vi "NI-XNET Frame&Log - CAN Frame to Table.vi"(1 "Hexadecimal?":bool, 5 "CAN Frames":T1[](array[typedef]) {"payload" format="%x"; "timestamp" format="%<%.7X\n%x>T"; "type" items=["CAN Data"=0, "CAN Remote"=1, "CAN Bus Error"=2, "Delay"=224, "Log Trigger"=225, "Start Trigger"=226]; "identifier" format="%x"}) -> (4 "Output Array":string[][](array[string]))   [LabVIEW 2014]
uses:
  <vilib>/xnet/xnet.llb/XNET Frame CAN.ctl
  <vilib>/xnet/xnet.llb/XNET Frame Type CAN.ctl
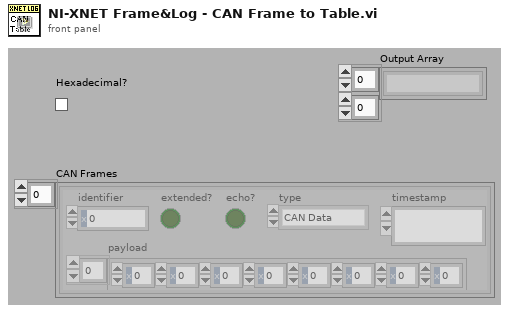
[diagram p1: front panel]
types:
  T1 = typedef "XNET Frame CAN.ctl" = cluster{"timestamp":timestamp, "payload":u8[], "identifier":u32, "type":T2, "extended?":bool, "echo?":bool}
  T2 = typedef "XNET Frame Type CAN.ctl" = u8
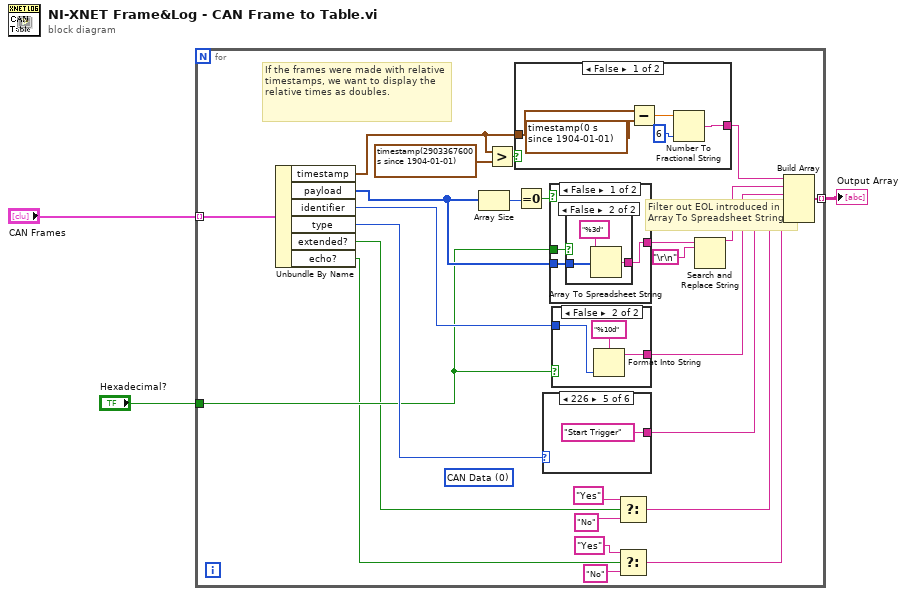
[diagram p0: block diagram]
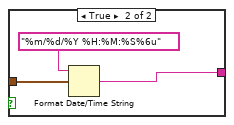
[diagram p2: hidden frame]
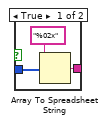
[diagram p3: hidden frame]
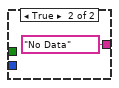
[diagram p4: hidden frame]
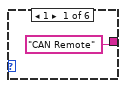
[diagram p5: hidden frame]
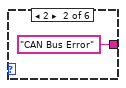
[diagram p6: hidden frame]
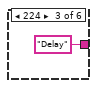
[diagram p7: hidden frame]
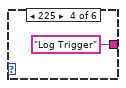
[diagram p8: hidden frame]
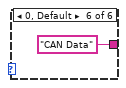
[diagram p9: hidden frame]
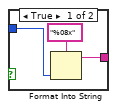
[diagram p10: hidden frame]
diagram:
  n1 = for {
    tunnel: "CAN Frames" -> [w28] mode=indexing
    tunnel: "Hexadecimal?" -> [w20]
    tunnel: [w19] -> w1 mode=indexing
    (unwired) T2 0 items=["CAN Data"=0, "CAN Remote"=1, "CAN Bus Error"=2, "Delay"=224, "Log Trigger"=225, "Start Trigger"=226] ("type")
    # "Filter out EOL introduced in \nArray To Spreadsheet String"
    # "If the frames were made with relative timestamps, we want to display the relative times as doubles."
    n2 = Unbundle By Name(w28) -> ("timestamp"=w10:timestamp, "payload"=w21:u8[], "identifier"=w27:u32, "type"=w25:T2, "extended?"=w12:bool, "echo?"=w18:bool)
    n3 = Array Size(array=w21) -> (size(s)=w23:i32)
    n4 = Greater?(x=w10, y=timestamp(2903367600 s since 1904-01-01)) -> (0:w7:bool)
    n5 = case shown="False" w7 {
      tunnel: w10 -> [w33 w35]
      tunnel: [w29 w34] -> w8
      frame False {
        n6 = Subtract(x=w33, y=timestamp(9.999999999615351e-10 s since 1904-01-01)) -> (x-y=w31:dbl)
        n7 = Number To Fractional String(number=w31, precision (6)=i16 6 ("width (-)")) -> (F-format string=w29:string)  [unwired: 2 out]
      }
      frame True {
        n8 = Format Date/Time String(time format string (%c)="%m/%d/%Y %H:%M:%S%6u", seconds (now)=w35) -> (date/time string=w34:string)  [unwired: 1 out]
      }
    }
    n9 = Equal To 0?(x=w23) -> (x = 0?=w22:bool)
    n10 = case shown="226" w25 {
      tunnel: ["CAN Remote" "CAN Bus Error" "Delay" "Log Trigger" "Start Trigger" "CAN Data"] -> w24
      frame 1 {
      }
      frame 2 {
      }
      frame 224 {
      }
      frame 225 {
      }
      frame 226 {
      }
      frame 0, Default {
      }
    }
    n11 = case shown="False" w22 {
      tunnel: [w37 "No Data"] -> w5
      tunnel: w21 -> [w39 _]
      tunnel: w20 -> [w38 _]
      frame False {
        n12 = case shown="False" w38 {
          tunnel: w39 -> [w41 w44]
          tunnel: [w40 w43] -> w37
          frame True {
            n13 = Array To Spreadsheet String(array=w41, 3:"%02x" ("format string")) -> (spreadsheet string=w40:string)  [unwired: 1 out]
          }
          frame False {
            n14 = Array To Spreadsheet String(array=w44, 3:"%3d" ("format string")) -> (spreadsheet string=w43:string)  [unwired: 1 out]
          }
        }
      }
      frame True {
      }
    }
    n15 = case shown="False" w20 {
      tunnel: w27 -> [w54 w57]
      tunnel: [w53 w56] -> w26
      frame True {
        n16 = Format Into String(format string="%08x", w54) -> (resulting string=w53:string)  [unwired: 2 in, 1 out]
      }
      frame False {
        n17 = Format Into String(format string="%10d", w57) -> (resulting string=w56:string)  [unwired: 2 in, 1 out]
      }
    }
    n18 = Select(t="Yes", s=w12, f="No") -> (s? t:f=w11:string)
    n19 = Select(t="Yes", s=w18, f="No") -> (s? t:f=w15:string)
    n20 = Search and Replace String(input string=w5, search string="\r\n") -> (result string=w4:string)  [unwired: 6 in, 3 out]
    n21 = Build Array(w8, w4, w26, w24, w11, w15) -> (w19:string[])
  }
  "Output Array" <- w1
